vi "OAXML_Block FFT.vi"(7 "Reset(F)":bool, 8 "window coefficients":dbl[](array[numeric]) format="%.2f", 11 "X":dbl[](array[numeric]) format="%.2f") -> (0 "Last Spectrum":cluster{"x[i]":dbl[], "y[i]":dbl[]} {"y[i]" format="%.2f"; "x[i]" format="%.2f"}, 3 "Block FFT Spectrum":dbl[][](array[numeric]) format="%.2f")   [LabVIEW 2017]
uses:
  <vilib>/Analysis/1siggen.llb/Ramp Pattern by Samples.vi
  <vilib>/Analysis/NI_AALPro.lvlib
  <vilib>/Analysis/NI_AALBase.lvlib
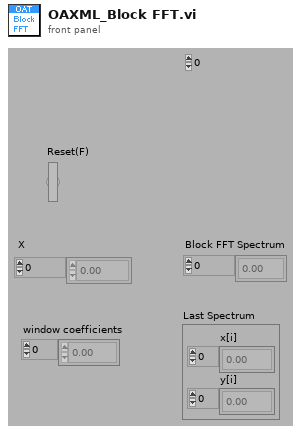
[diagram p1: front panel]
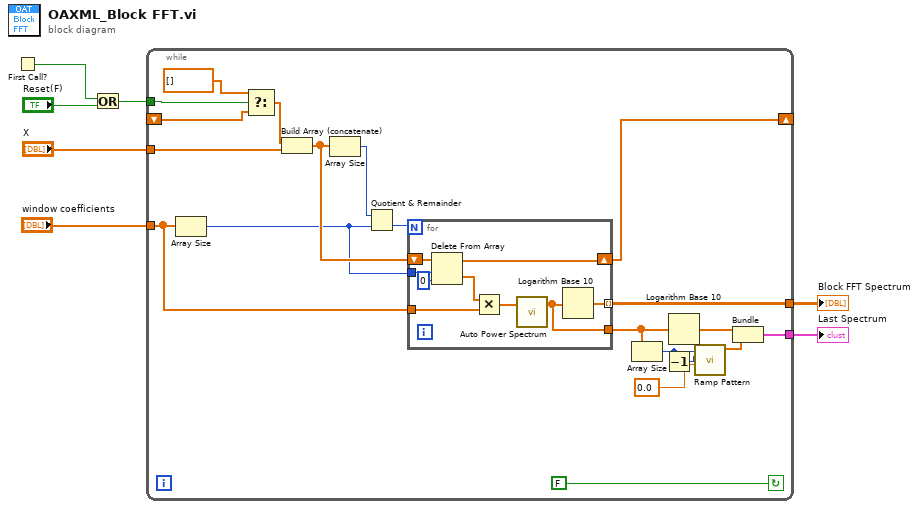
[diagram p0: block diagram]
diagram:
  n1 = First Call?() -> (First Call?: T/F=w6:bool)
  n2 = Or(x=w6, y="Reset(F)") -> (x .or. y?=w5:bool)
  n3 = while {
    shift-right: [w17] -> _
    shift-left: _ -> [w24]
    tunnel: w5 -> [w26]
    tunnel: "X" -> [w23]
    tunnel: "window coefficients" -> [w16]
    tunnel: [w15] -> w2
    tunnel: [w10] -> w1
    stop <- FALSE continue-if-true
    n4 = Array Size(array=w16) -> (size(s)=w18:i32)
    n5 = Select(t=sgl[] [], s=w26, f=w24) -> (s? t:f=w22:dbl[])
    n6 = Build Array (concatenate)(w22, w23) -> (w19:dbl[])
    n7 = Array Size(array=w19) -> (size(s)=w21:i32)
    n8 = Quotient & Remainder(x=w21, y=w18) -> (floor(x/y)=w20:i32)  [unwired: 1 out]
    n9 = for {
      N: w20 -> [_]
      shift-right: [w34] -> w17
      shift-left: w19 -> [w36]
      tunnel: w18 -> [w35]
      tunnel: w16 -> [w33]
      tunnel: [w31] -> w15 mode=indexing
      tunnel: [w30] -> w9
      n10 = Delete From Array(array=w36, length=w35, index=0) -> (deleted portion=w29:dbl[], array with subset deleted=w34:dbl[])
      n11 = Multiply(x=w29, y=w33) -> (x*y=w32:dbl[])
      n12 = call <vilib>:"Auto Power Spectrum.vi"("Signal (V)"=w32) -> ("Power Spectrum (V^2 rms)"=w30:dbl[])  [unwired: 1 in, 1 out]
      n13 = Logarithm Base 10(1:w30) -> (0:w31:dbl[])
    }
    n14 = Array Size(array=w9) -> (size(s)=w11:i32)
    n15 = Decrement(x=w11) -> (x-1=w12:i32)
    n16 = Logarithm Base 10(1:w9) -> (0:w8:dbl[])
    n17 = call-poly <vilib>:"Ramp Pattern.vi"("start"=0.0, "end"=w12, "samples"=w11) -> ("Ramp Pattern"=w14:dbl[])  [unwired: 7 in, 1 out]
    n18 = Bundle(w8, "Ramp Pattern"=w14) -> (w10:cluster{dbl[], "Ramp Pattern":dbl[]})  [unwired: 1 in]
  }
  "Block FFT Spectrum" <- w2
  "Last Spectrum" <- w1
